vi "Close Sample Container Connections.vi"(8 "error in (no error)":errorcluster, 11 "Syringe in":refnum<class "Syringe Line.lvclass">) -> (0 "error out":errorcluster, 3 "Syringe out":refnum<class "Syringe Line.lvclass">)   [LabVIEW 2015, in "cRIO-Carbondioxide.lvlib" / "CO2-Actor.lvlib" / "Syringe Line.lvclass"]
uses:
  Syringe Line.lvclass
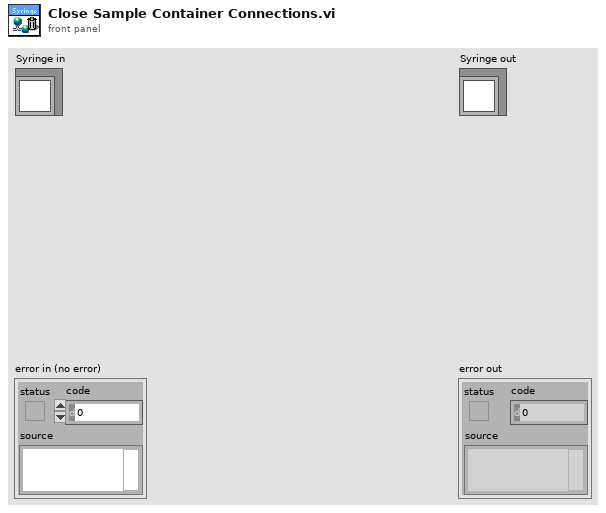
[diagram p1: front panel]
types:
  T1 = typedef "Sample Container.ctl" = cluster{"Sample In":refnum<k21>, "Sample Name":refnum<k21>, "Ti Cathode":refnum<k21>, "SampleQ":refnum<queue>}
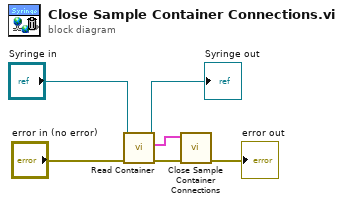
[diagram p0: block diagram]
diagram:
  n1 = call "Read Container.vi"("error in (no error)"="error in (no error)", "Syringe Line in"="Syringe in") -> ("error out"=w4:errorcluster, "Container"=w1:T1, "Syringe Line out"=→"Syringe out":refnum<class "Syringe Line.lvclass">)  [unwired: 6 in, 1 out]
  n2 = call "Close Sample Container Connections.vi"("error in (no error)"=w4, "Container in"=w1) -> ("error out"=→"error out":errorcluster)  [unwired: 8 in, 1 out]
